vi "Frame Calc Insert.vi"(1 "Array Size":u32, 3 "ActualEntry":u32, 5 "Tlg Data Array":T2 {"CAN frame In"."FlexRay"."cycle count" max=63 step=1; "CAN frame In"."payload" format="%x"; "CAN frame In"."identifier / slot" format="%x"; "FlexRay Channel" items=["A", "B", "A+B"]}, 6 "Actual Read frame":T1={"timestamp"=timestamp(0 s since 1904-01-01), "payload"=[0, 0, 0, 0, 0, 0, 0, 0], "identifier / slot"=0, "Data type"=0, "payload length"=0, "CAN"={"extended?"=FALSE}, "FlexRay"={"cycle count"=0, "startup?"=FALSE, "sync?"=FALSE, "preamble?"=FALSE, "ch A"=FALSE, "ch B"=FALSE, "macrotick"=32}, "echo?"=FALSE} {"FlexRay"."cycle count" max=63 step=1; "payload" format="%x"; "identifier / slot" format="%x"}) -> (0 "Tlg Data Array Out":T2 {"CAN frame In"."FlexRay"."cycle count" max=63 step=1; "CAN frame In"."payload" format="%x"; "CAN frame In"."identifier / slot" format="%x"; "FlexRay Channel" items=["A", "B", "A+B"]})   [LabVIEW 2014, in "CAN Bus Monitor Engine.lvlib"]
uses:
  CAN Bus Monitor Engine.lvlib
  Controls/Analyze Array.ctl
  Controls/FlexRay Channel.ctl
  Controls/XNET BM Frame.ctl
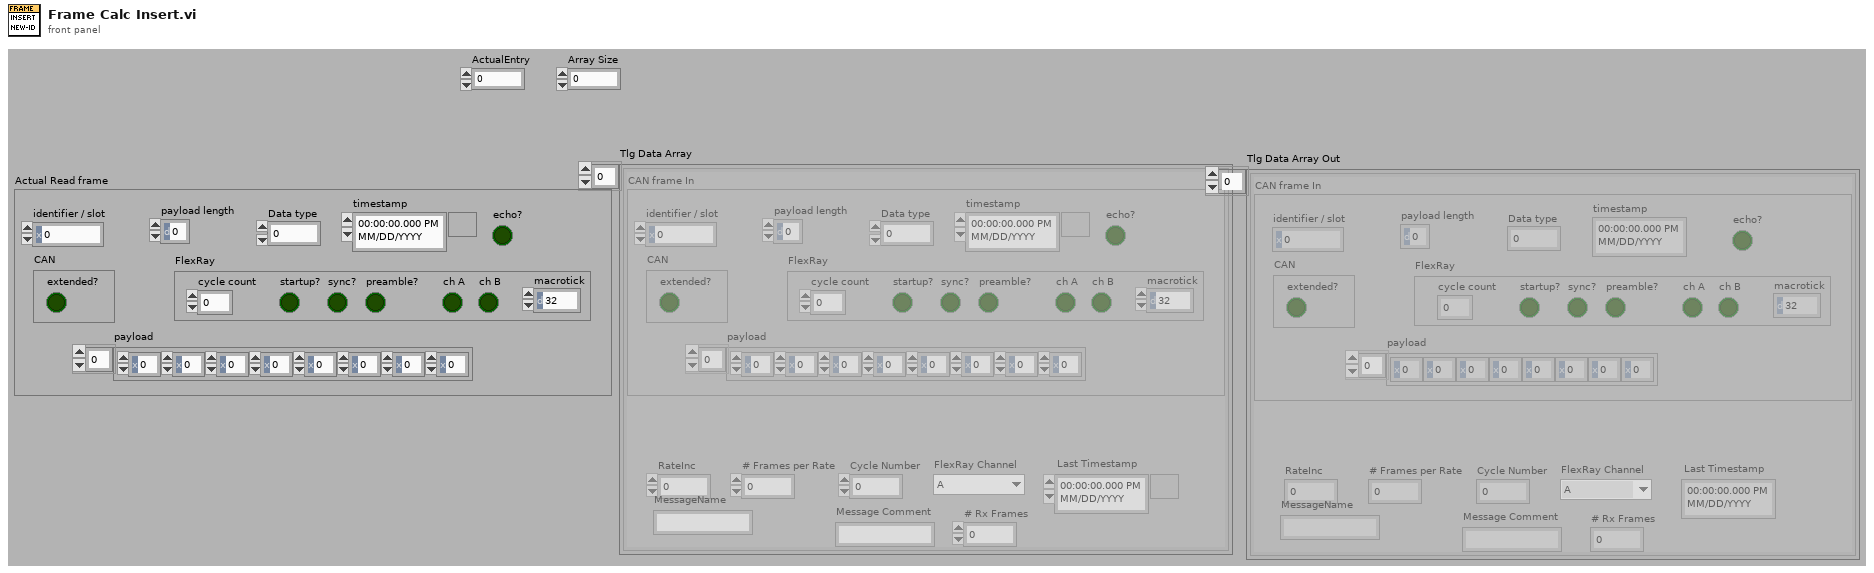
[diagram p1: front panel]
types:
  T1 = typedef "CAN Bus Monitor Engine.lvlib/XNET BM Frame.ctl" = cluster{"timestamp":timestamp, "payload":u8[], "identifier / slot":u32, "Data type":u8, "payload length":u8, "CAN":cluster{"extended?":bool}, "FlexRay":cluster{"cycle count":u8, "startup?":bool, "sync?":bool, "preamble?":bool, "ch A":bool, "ch B":bool, "macrotick":u16}, "echo?":bool}
  T2 = typedef "CAN Bus Monitor Engine.lvlib/Analyze Array.ctl" = cluster{"# Rx Frames":u32, "Last Timestamp":timestamp, "RateInc":dbl, "# Frames per Rate":u32, "MessageName":string, "Cycle Number":u32, "FlexRay Channel":T3, "Message Comment":string, "CAN frame In":T1}[]
  T3 = typedef "CAN Bus Monitor Engine.lvlib/FlexRay Channel.ctl" = u16
  T4 = cluster{"# Rx Frames":u32, "Last Timestamp":timestamp, "RateInc":dbl, "# Frames per Rate":u32, "MessageName":string, "Cycle Number":u32, "FlexRay Channel":T3, "Message Comment":string, "CAN frame In":T1}
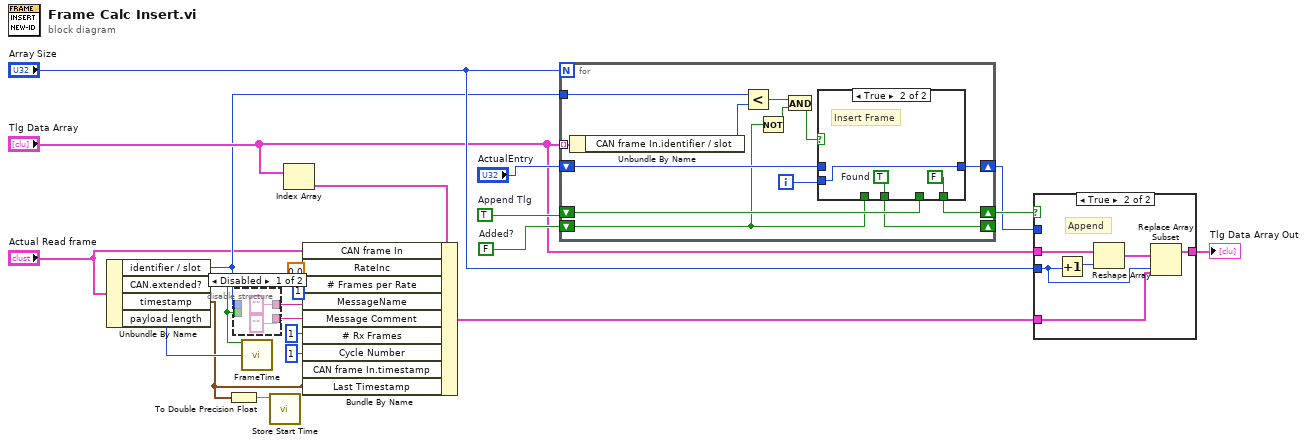
[diagram p0: block diagram]
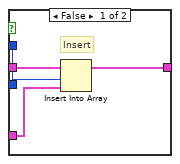
[diagram p3: hidden frame]
diagram:
  w13 = FALSE  # Added?
  w19 = TRUE  # Append Tlg
  n1 = Unbundle By Name("Actual Read frame") -> ("identifier / slot"=w7:u32, "CAN.extended?"=w5:bool, "timestamp"=w2:timestamp, "payload length"=w4:u8)
  n2 = To Double Precision Float(number=w2) -> (double precision float=w3:dbl)
  n3 = disable-structure shown="Disabled" {
    disable-tunnel: ["" ("MessageName") _] -> w14
    disable-tunnel: ["" ("MessageComment") _] -> w11
    disable-tunnel: w7 -> [_ _]
    disable-tunnel: w5 -> [_ _]
    frame Disabled {
    }
    frame Enabled {
    }
  }
  n4 = call "FrameTime.vi"("Is Extended ID?"=w5, "DataLength"=w4) -> ()  [unwired: 14 in]
  n5 = call "Store Start Time.vi"("Timestamp"=w3) -> ()  [unwired: 11 in]
  n6 = Index Array(array="Tlg Data Array") -> (element=w9:T4)  [unwired: 1 in]
  n7 = Bundle By Name(cluster=w9, "CAN frame In"="Actual Read frame", "RateInc"=0.0, "# Frames per Rate"=u32 1, "MessageName"=w14, "Message Comment"=w11, "# Rx Frames"=u32 1 ("# of Frames"), "Cycle Number"=u32 1 ("# of Frames"), "CAN frame In.timestamp"=w2, "Last Timestamp"=w2) -> (w8:T4)
  n8 = for {
    N: "Array Size" -> [_]
    tunnel: "Tlg Data Array" -> [w35] mode=indexing
    tunnel: w7 -> [w36]
    shift-right: [w32] -> w17
    shift-left: "ActualEntry" -> [w33]
    shift-right: [w30] -> w18
    shift-left: w19 -> [w31]
    shift-right: [w29] -> _
    shift-left: w13 -> [w27]
    i -> [w34]
    n9 = Unbundle By Name(w35) -> ("CAN frame In.identifier / slot"=w37:u32)
    n10 = Less?(x=w36, y=w37) -> (x < y?=w26:bool)
    n11 = Not(x=w27) -> (.not. x?=w28:bool)
    n12 = And(x=w26, y=w28) -> (x .and. y?=w25:bool)
    n13 = case shown="True" w25 {
      tunnel: w34 -> [_ w41]
      tunnel: [w40 w41] -> w32
      tunnel: w33 -> [w40 _]
      tunnel: w31 -> [w38 _]
      tunnel: [w38 FALSE ("Append Tlg")] -> w30
      tunnel: [w39 w43] -> w29
      tunnel: w27 -> [w39 _]
      frame False {
      }
      frame True {
        w43 = TRUE  # Found
        # "Insert Frame"
      }
    }
  }
  n14 = case shown="True" w18 {
    tunnel: "Tlg Data Array" -> [w47 w53]
    tunnel: w17 -> [w45 _]
    tunnel: [w46 w51] -> w20
    tunnel: "Array Size" -> [_ w49]
    tunnel: w8 -> [w44 w48]
    frame False {
      # "Insert"
      n15 = Insert Into Array(array=w47, index=w45, new element=w44) -> (w46:T2)
    }
    frame True {
      # "Append"
      n16 = Increment(x=w49) -> (x+1=w50:u32)
      n17 = Reshape Array(w53, w50) -> (w52:T2)
      n18 = Replace Array Subset(array=w52, new element=w48, index=w49) -> (w51:T2)
    }
  }
  "Tlg Data Array Out" <- w20
